vi "FiberSpectrograph_acceptCommand_setSimulationMode.vi"(8 "error in (no error)":errorcluster, 11 "command_setSimulationMode_Ctl":T1) -> (0 "error out":errorcluster, 2 "function return":i32, 3 "command_setSimulationMode_Ctl out":T1)   [LabVIEW 2016, in "SALLV_FiberSpectrograph.lvlib"]
doc: "int FiberSpectrograph_shm_acceptCommand_setSimulationModeLV(FiberSpectrograph_command_setSimulationModeLV *command_setSimulationMode_Ctl );"
uses:
  SALLV_FiberSpectrograph.lvlib
  DataTypes/command_setSimulationMode.ctl
  SALLV_FiberSpectrograph.so
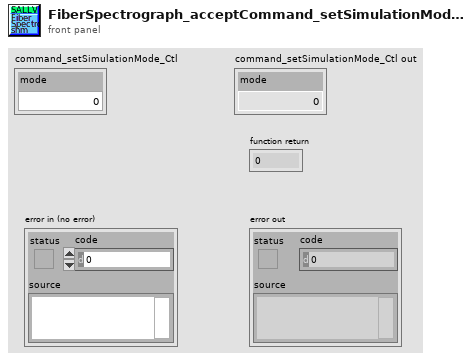
[diagram p1: front panel]
types:
  T1 = typedef "SALLV_FiberSpectrograph.lvlib/command_setSimulationMode.ctl" = cluster{"mode":i32}
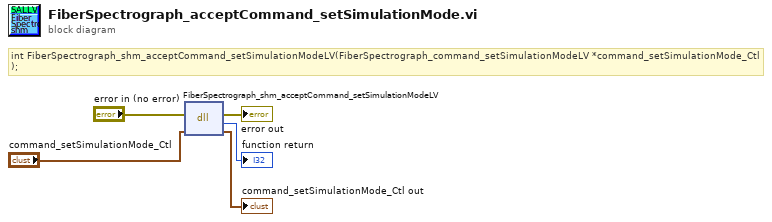
[diagram p0: block diagram]
diagram:
  # "int FiberSpectrograph_shm_acceptCommand_setSimulationModeLV(FiberSpectrograph_command_setSimulationModeLV *command_setSimulationMode_Ctl );"
  n1 = dll-call lib="home/harini/SALLV_FiberSpectrograph/SALLV_FiberSpectrograph.*" fn="FiberSpectrograph_shm_acceptCommand_setSimulationModeLV"(error in="error in (no error)", "command_setSimulationMode_Ctl"="command_setSimulationMode_Ctl") -> (error out=→"error out":errorcluster, →"function return":i32, "command_setSimulationMode_Ctl"=→"command_setSimulationMode_Ctl out":T1)  [unwired: 2 in, 1 out]
